vi "oa_Check dr of Multi Channel Signals.vi"(2 "error in (no error)":errorcluster, 3 "even angle signals in":cluster{"r0":dbl, "dr":dbl, "Y":dbl[]}[](array[cluster]) {"r0" format="%.2p"; "dr" format="%.2p"; "Y" format="%.2f"}) -> (0 "error out":errorcluster, 1 "even angle signals out":cluster{"r0":dbl, "dr":dbl, "Y":dbl[]}[](array[cluster]) {"r0" format="%.2p"; "dr" format="%.2p"; "Y" format="%.2f"})   [LabVIEW 2017, in "SoundVib_OAUtility.lvlib"]
uses:
  <vilib>/addons/Sound and Vibration/Order Analysis/Utility/SoundVib_OAUtility.lvlib
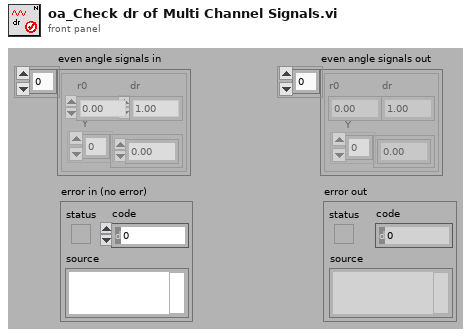
[diagram p1: front panel]
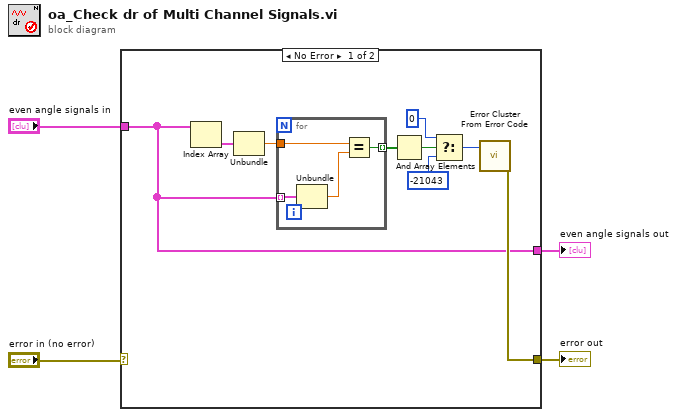
[diagram p0: block diagram]
diagram:
  n1 = case shown="No Error" "error in (no error)" {
    selector: "error in (no error)" -> [_ w19]
    tunnel: "even angle signals in" -> [w5 w18]
    tunnel: [w6 w19] -> w2
    tunnel: [w5 w18] -> w1
    frame No Error {
      n2 = Index Array(array=w5) -> (element=w13:cluster{"r0":dbl, "dr":dbl, "Y":dbl[]})  [unwired: 1 in]
      n3 = Unbundle(w13) -> ("dr"=w12:dbl)  [unwired: 2 out]
      n4 = for {
        tunnel: w12 -> [w16]
        tunnel: w5 -> [w17] mode=indexing
        tunnel: [w14] -> w11 mode=indexing
        n5 = Unbundle(w17) -> ("dr"=w15:dbl)  [unwired: 2 out]
        n6 = Equal?(x=w16, y=w15) -> (x = y?=w14:bool)
      }
      n7 = And Array Elements(Boolean array=w11) -> (logical AND=w10:bool)
      n8 = Select(t=0, s=w10, f=-21043) -> (s? t:f=w7:i32)
      n9 = call <vilib>:"Error Cluster From Error Code.vi"("error code (0)"=w7) -> ("error out"=w6:errorcluster)  [unwired: 8 in]
    }
    frame Error {
    }
  }
  "error out" <- w2
  "even angle signals out" <- w1
